vi "dns-pid identifier string.vi"() -> (0 "DNS_PID Identifier string":string)   [LabVIEW 2017]
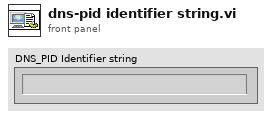
[diagram p1: front panel]
types:
  T1 = enum32{"invalid app kind", "Development System", "Run Time System", "Student Edition", "Embedded LabVIEW", "Evaluation", "Custom"}
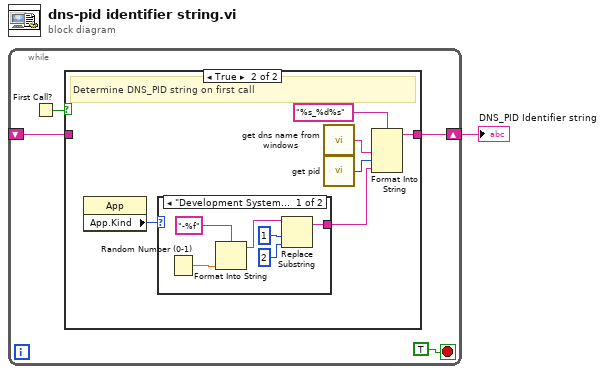
[diagram p0: block diagram]
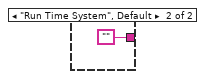
[diagram p3: hidden frame]
diagram:
  n1 = while {
    shift-right: [w3] -> w1
    shift-left: _ -> [w2]
    stop <- TRUE stop-if-true
    n2 = First Call?() -> (First Call?: T/F=w4:bool)
    n3 = case shown="True" w4 {
      tunnel: [w6 w7] -> w3
      tunnel: w2 -> [w6 _]
      frame False {
        # "Serve previously generated string"
      }
      frame True {
        # "Determine DNS_PID string on first call"
        n4 = property class="App"() -> ("App.Kind"=w11:T1)  [unwired: 2 in, 2 out]
        n5 = case shown="\"Development System\"" w11 {
          tunnel: [w13 ""] -> w12
          frame "Development System" {
            n6 = Random Number (0-1)() -> (number: 0 to 1=w17:dbl)
            n7 = Format Into String(format string="-%f", w17) -> (resulting string=w18:string)  [unwired: 2 in, 1 out]
            n8 = Replace Substring(2:2 ("length (len. of substring)"), 3:1 ("offset (0)"), 5:w18) -> (1:w13:string)  [unwired: 1 in, 1 out]
          }
          frame "Run Time System", Default {
          }
        }
        n9 = call "get dns name from windows.vi"() -> ("ToString"=w9:string)  [unwired: 1 in]
        n10 = call "get pid.vi"() -> ("PID"=w10:u32)  [unwired: 1 in]
        n11 = Format Into String(format string="%s_%d%s", w9, w10, w12) -> (resulting string=w7:string)  [unwired: 2 in, 1 out]
      }
    }
  }
  "DNS_PID Identifier string" <- w1
